vi "CAN task.vi"(7 "CANopen in":refnum<class "CANopen.lvclass">) -> ()   [LabVIEW 2024, in "canopen.lvlib" / "CANopen.lvclass"]
doc: "Starts the task that reads messages and tries to handle them."
uses:
  CANopen.lvclass
  CANopen.lvclass/CANopen.ctl
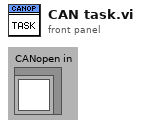
[diagram p1: front panel]
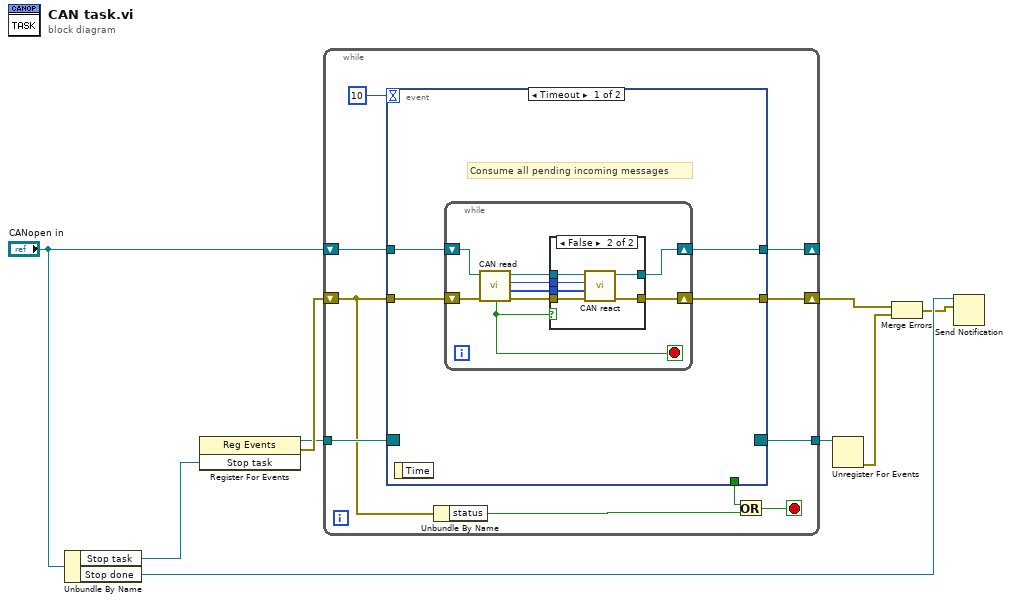
[diagram p0: block diagram]
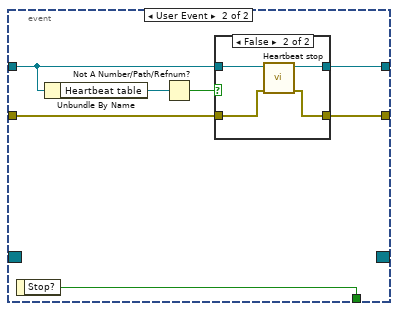
[diagram p3: hidden frame]
diagram:
  n1 = Unbundle By Name("CANopen in") -> ("Stop task"=w3:refnum<user-event>, "Stop done"=w5:refnum<notifier>)
  n2 = register-events(w3) -> (reference out=w8:refnum<event-registration>, error out=w9:errorcluster)  [unwired: 2 in]
  n3 = while {
    shift-right: [w19] -> w2
    shift-left: w9 -> [w15]
    tunnel: w8 -> [w17]
    tunnel: [w16] -> w7
    shift-right: [w10] -> _
    shift-left: "CANopen in" -> [w11]
    stop <- w14 stop-if-true
    n4 = event shown="[0] Timeout" {
      selector: w17 -> [_ _]
      dyn-events: [_ _] -> w16
      timeout: 10 -> [_ _]
      tunnel: [_ w47] -> w13
      tunnel: [w23 w44] -> w19
      tunnel: w15 -> [w21 w45]
      tunnel: w11 -> [w20 w43]
      tunnel: [w22 w46] -> w10
      event Timeout {
        # "Consume all pending incoming messages"
        n5 = event-data() -> ()  [unwired: 2 out]
        n6 = while {
          shift-right: [w32] -> w23
          shift-left: w21 -> [w30]
          shift-right: [w31] -> w22
          shift-left: w20 -> [w27]
          stop <- w24 stop-if-true
          n7 = call "CAN read.vi"("error in (no error)"=w30, "CANopen in"=w27) -> ("error out"=w29:errorcluster, "Data"=w25:u8[], "COB id"=w26:i32, "CANopen out"=w28:refnum<class "CANopen.lvclass">, "No data?"=w24:bool)  [unwired: 3 out]
          n8 = case shown="False" w24 {
            tunnel: w29 -> [w34 w40]
            tunnel: [w34 w39] -> w32
            tunnel: [w33 w37] -> w31
            tunnel: w28 -> [w33 w38]
            tunnel: w26 -> [_ w35]
            tunnel: w25 -> [_ w36]
            frame True {
            }
            frame False {
              n9 = call "CAN react.vi"("error in (no error)"=w40, "Data"=w36, "COB id"=w35, "CANopen in"=w38) -> ("error out"=w39:errorcluster, "CANopen out"=w37:refnum<class "CANopen.lvclass">)  [unwired: 2 out]
            }
          }
        }
      }
      event User Event {
        n10 = event-data() -> ("Stop?"=w47:bool)  [unwired: 1 out]
        n11 = Unbundle By Name(w43) -> ("Heartbeat table"=w42:refnum<vi>)
        n12 = Not A Number/Path/Refnum?(number/path/refnum=w42) -> (NaN/Path/Refnum?=w41:bool)
        n13 = case shown="False" w41 {
          tunnel: [w49 w53] -> w46
          tunnel: w45 -> [w48 w52]
          tunnel: [w48 w51] -> w44
          tunnel: w43 -> [w49 w50]
          frame True {
          }
          frame False {
            n14 = call "Heartbeat stop.vi"("error in"=w52, "CANopen in"=w50) -> ("error out"=w51:errorcluster, "CANopen out"=w53:refnum<class "CANopen.lvclass">)  [unwired: 1 in, 3 out]
          }
        }
      }
    }
    n15 = Unbundle By Name(w15) -> ("status"=w12:bool)
    n16 = Or(x=w13, y=w12) -> (x .or. y?=w14:bool)
  }
  n17 = Unregister For Events(event registration refnum=w7) -> (error out=w1:errorcluster)  [unwired: 1 in]
  n18 = Merge Errors(w2, w1) -> (w4:errorcluster)
  n19 = Send Notification(notification=w4, notifier=w5) -> ()  [unwired: 1 in, 2 out]
